vi "command_center.vi"(0 "reference (in)":i32=4168, 5 "commands":T1[](array[typedef]), 7 "data (in)":string, 11 "error in (no error)":errorcluster) -> (4 "reference (out)":i32=4168, 8 "data (out)":string, 15 "error out":errorcluster)   [LabVIEW 2012]
doc: "This is an EXAMPLE of a piece of code one might implement to call multiple commands to the hardware referneced by the reference value passed in. Note, however, if more than one command in the array of commands to be called contains a parameter as input, the developer MUST account for this in the calling VI. Although this VI is capable of supporting optional command parameters, it is otherwise best used to call consecutive commands that do not contain parameters.\n\nProduced By:\n\nChristopher Lemieux\nKod Integrations, LLC\n4835 Marianne Drive\nMount Airy, MD 21771\nhttp://www.kodintegrations.com\nemail: clemieux@kodintegrations.com\nphone: (240) 687-1288"
uses:
  main_functions/commands.ctl
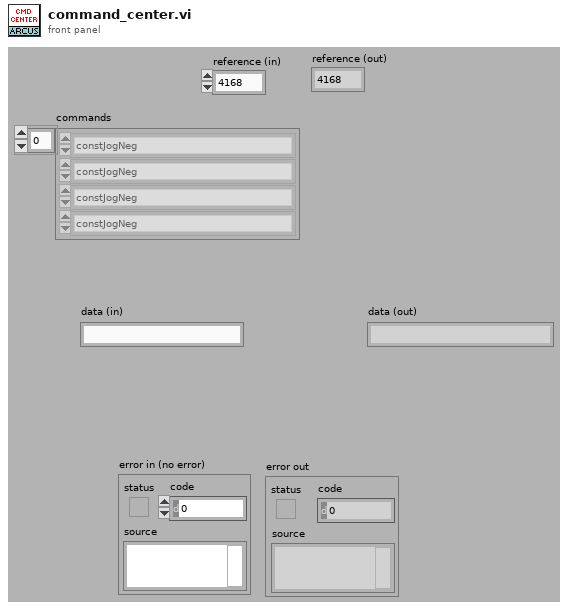
[diagram p1: front panel]
types:
  T1 = typedef "commands.ctl" = enum16{"clearErr", "constJogNeg", "constJogPos", "getAccel", "getActualAmp", "getDeviceId", "getDigInputStatus", "getDigInputsStatus", "getDigOutputStatus", "getDigOutputsStatus", "getFirmwareVer", "getHighSpeed", "getIdleAmp", "getLowSpeed", "getMicroStep", "getMotorStatus", "getMoveMode", "getPolarity", "getPosition", "getProdId", "getPwrStatus", "getRunAmp", "getStatus", "homeNeg", "homePos", "moveToPosition", "powerDown", "powerUp", "setAccel", "setDeviceId", "setDigOutput", "setDigOutputs", "setHighSpeed", "setIdleAmp", "setLowSpeed", "setMoveModeAbs", "setMoveModeIncr", "setPolarity", "setPosition", "setRunAmp", "stopNow", "stopSlow", "storeToMem"}
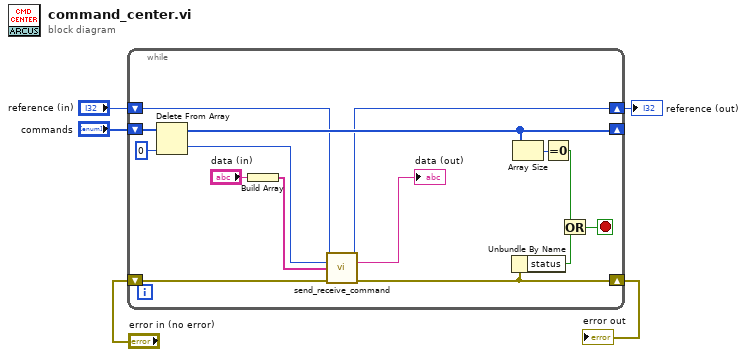
[diagram p0: block diagram]
diagram:
  n1 = while {
    shift-right: [w17] -> _
    shift-left: "commands" -> [w20]
    shift-right: [w14] -> w3
    shift-left: "error in (no error)" -> [w16]
    shift-right: [w9] -> w1
    shift-left: "reference (in)" -> [w10]
    stop <- w11 stop-if-true
    n2 = Delete From Array(array=w20, index=0) -> (deleted portion=w18:T1, array with subset deleted=w17:T1[])  [unwired: 1 in]
    n3 = Build Array("data (in)") -> (w6:string[])
    n4 = call "send_receive_command.vi"("reference (in)"=w10, "command"=w18, "params (opt)"=w6, "error in (no error)"=w16) -> ("reference (dup)"=w9:i32, "read_string"=→"data (out)":string, "error out"=w14:errorcluster)  [unwired: 7 in, 2 out]
    n5 = Unbundle By Name(w14) -> ("status"=w12:bool)
    n6 = Array Size(array=w17) -> (size(s)=w15:i32)
    n7 = Equal To 0?(x=w15) -> (x = 0?=w13:bool)
    n8 = Or(x=w13, y=w12) -> (x .or. y?=w11:bool)
  }
  "error out" <- w3
  "reference (out)" <- w1
